vi "practica12.vi"() -> ()   [LabVIEW 2016]
panel:
  out "a 3":dbl
  in  "w 3":dbl[](array[numeric])
  in  "b 3":dbl
  in  "w 2":dbl[](array[numeric])
  in  "b 2":dbl
  in  "b":dbl
  in  "w":dbl[](array[numeric])
  in  "x":dbl[](array[numeric])
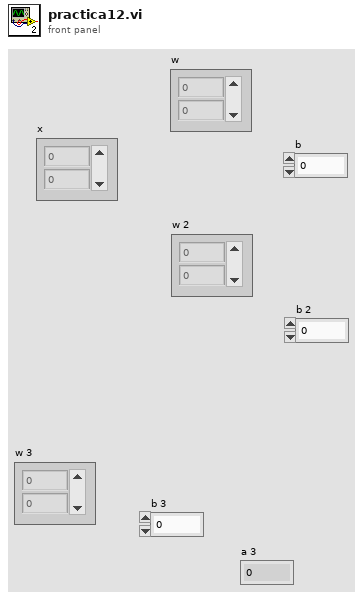
[diagram p1: front panel]
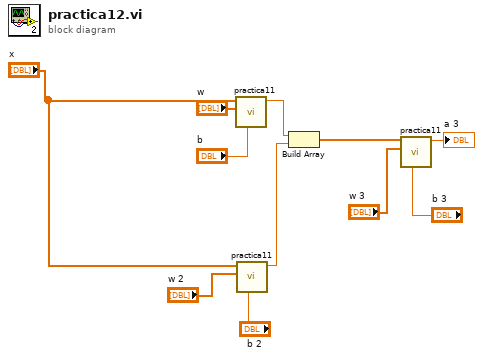
[diagram p0: block diagram]
diagram:
  n1 = call "practica11.vi"("b"="b", "w"="w", "x"="x") -> ("a"=w1:dbl)  [unwired: 8 in]
  n2 = call "practica11.vi"("b"="b 2", "w"="w 2", "x"="x") -> ("a"=w5:dbl)  [unwired: 8 in]
  n3 = Build Array(w1, w5) -> (w4:dbl[])
  n4 = call "practica11.vi"("b"="b 3", "w"="w 3", "x"=w4) -> ("a"=→"a 3":dbl)  [unwired: 8 in]
